vi "Create Live Random Data.vi"(0 "Input AnchorArray":refnum<class "Anchor.lvclass">[](array[class]), 7 "Tag.lvclass":refnum<class "Tag.lvclass">, 11 "Input":T3) -> (4 "PositionOut":T1, 8 "Output AnchorArray":refnum<class "Anchor.lvclass">[](array[class]), 15 "Output Tag":refnum<class "Tag.lvclass">)   [LabVIEW 2014]
doc: "This VI create random generated data based on its previous input, an array of Anchor objects and a single Tag object which we want its position estimated. The VI returns the Tag id, estimated position, and the altered array of Anchor objects. DistanceLimit control manages the limit on measured distances. If the measured distance >= DistanceLimit the distance is set to an invalid number so it will not be taken into account for position estimation. This control serves to simulate real world scenario where a signal can be lost\nafter a certain amount of meters."
uses:
  Tag.lvclass
  Anchor/Anchor.lvclass
panel:
  in  "DistanceLimit":dbl=90.0
  out "Tag out":refnum<class "Tag.lvclass">
  out "error out 2":errorcluster
  in  "error in (no error) 2":errorcluster
  out "error out":errorcluster
  in  "error in (no error)":errorcluster
  out "AnchorIDDistanceCluster":T2
  out "NumberOfAnchors":i32
  out "AnchorClusterArray":T4(array[cluster])
  out "TagY":dbl
  out "TagX":dbl
  out "TagID":dbl
  out "x rand":dbl
  out "y rand":dbl
  out "Start y":dbl=30.0
  out "Start x":dbl=61.0
  # "Use dynamic anchor array for multiple anchors.\nStandard is 3 anchors."
  # "Result of Create Random XY VI\nCompare with output for analysis"
  # "[tagID, x, y, anchorID, distances]"
  # "tagID, X, Y, [anchorID, distance]"
  # "Tag which has updated XY values"
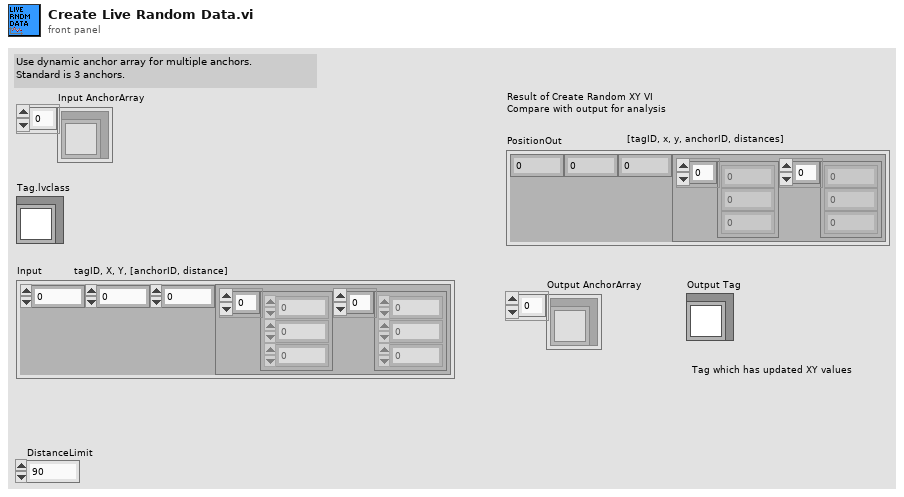
[diagram p1: front panel]
types:
  T1 = cluster{"tagID":dbl, "X":dbl, "Y":dbl, "anchorIDDistanceCluster":cluster{"anchorIDArray":dbl[], "anchorDistanceArray":dbl[]}}
  T2 = cluster{"AnchorIDArrayConstant":dbl[], "AnchorDistanceConstant":dbl[]}
  T3 = cluster{"Tag":dbl, "X":dbl, "Y":dbl, "AnchorIDDistanceCluster":cluster{"AnchorIDArray":dbl[], "AnchorDistancesArray":dbl[]}}
  T4 = cluster{"AnchorID":dbl, "AnchorX":dbl, "AnchorY":dbl}[]
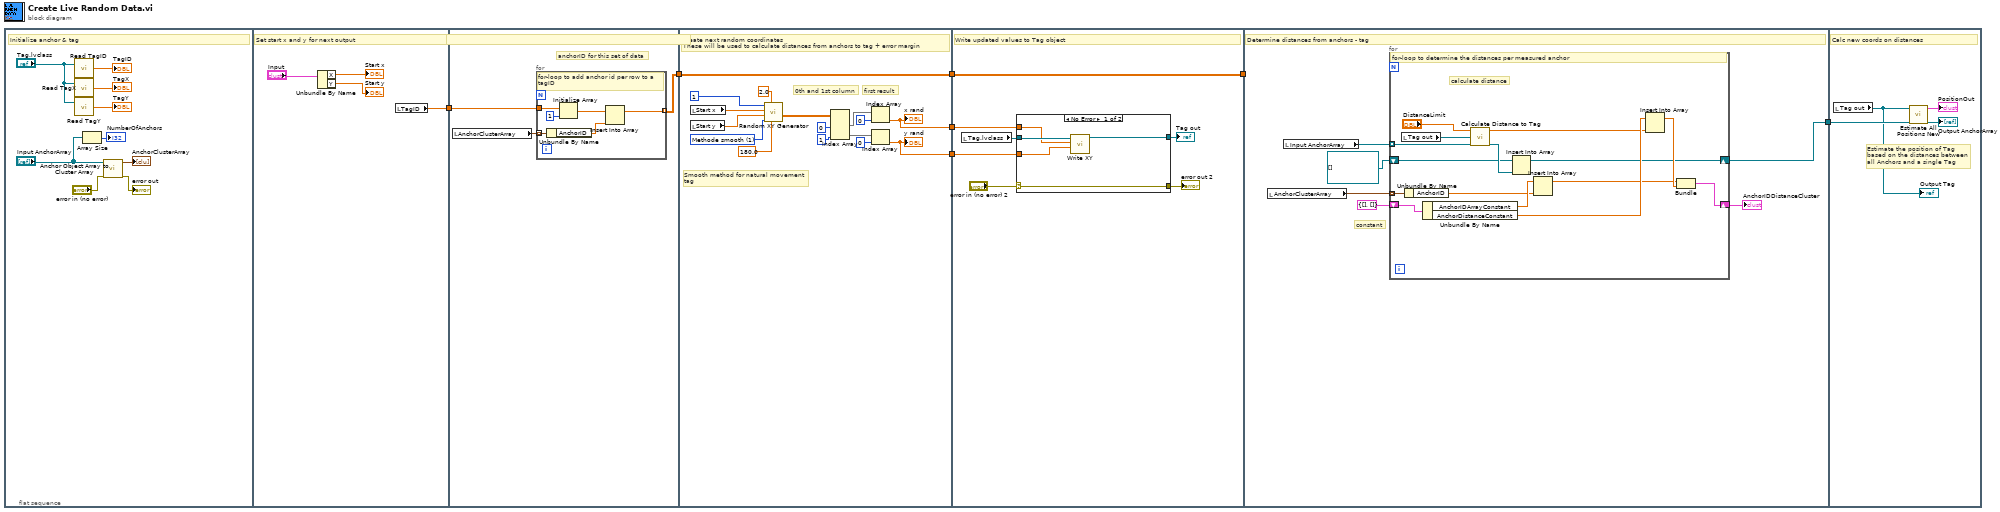
[diagram p0: block diagram]
diagram:
  n1 = flat-sequence {
    tunnel: [w20] -> w6
    tunnel: [w21] -> w7
    tunnel: w6 -> [w23]
    tunnel: [w45] -> w4
    tunnel: w7 -> [w45]
    tunnel: [w31] -> w2
    tunnel: [w30] -> w1
    tunnel: w4 -> [w52]
    tunnel: [w52] -> w3
    tunnel: w2 -> [w50]
    tunnel: w1 -> [w49]
    tunnel: w3 -> [_]
    tunnel: [w60] -> w5
    tunnel: w5 -> [w84]
    frame #0 {
      # "Initialize anchor & tag"
      n2 = call-dynamic "Read TagID.vi"("Tag in"="Tag.lvclass") -> ("TagID"=→"TagID":dbl)  [unwired: 1 in, 2 out]
      n3 = call-dynamic "Read TagX.vi"("Tag in"="Tag.lvclass") -> ("TagX"=→"TagX":dbl)  [unwired: 1 in, 2 out]
      n4 = call-dynamic "Read TagY.vi"("Tag in"="Tag.lvclass") -> ("TagY"=→"TagY":dbl)  [unwired: 1 in, 2 out]
      n5 = Array Size(array="Input AnchorArray") -> (size(s)=→"NumberOfAnchors":i32)
      n6 = call "Anchor Object Array to Cluster Array.vi"("error in (no error)"="error in (no error)", "AnchorArray In"="Input AnchorArray") -> ("error out"=→"error out":errorcluster, "AnchorArray Out"=→"AnchorClusterArray":T4)  [unwired: 8 in]
    }
    frame #1 {
      # "Set start x and y for next output"
      n7 = Unbundle By Name("Input") -> ("X"=→"Start x":dbl, "Y"=→"Start y":dbl)
      n8 = local read "TagID"() -> (w20:dbl)
    }
    frame #2 {
      # "anchorID for this set of data"
      # "Create anchor IDs"
      n9 = local read "AnchorClusterArray"() -> (w22:T4)
      n10 = for {
        tunnel: w23 -> [w28]
        tunnel: w22 -> [w29] mode=indexing
        tunnel: [w24] -> w21 mode=indexing
        # "for-loop to add anchor id per row to a tagID"
        n11 = Unbundle By Name(w29) -> ("AnchorID"=w25:dbl)
        n12 = Initialize Array ("Initialize Tag ID Row Array")(w28, 1 ("dimension size")) -> (w26:dbl[])
        n13 = Insert Into Array(array=w26, new element=w25) -> (w24:dbl[])  [unwired: 1 in]
      }
    }
    frame #3 {
      w44 = u16 1 items=["Methode Random", "Methode smooth"] ("Random Methode")
      # "first result"
      # "0th and 1st column"
      # "Smooth method for natural movement\ntag"
      # "Create next random coordinates\nThese will be used to calculate distances from anchors to tag + error margin"
      n14 = local read "Start x"() -> (w42:dbl)
      n15 = local read "Start y"() -> (w43:dbl)
      n16 = call "Random XY Generator.vi"("MaxHeading"=180.0 ("Max h variatie"), "MaxVelocity"=2.0 ("Max V variatie"), "Random Methode"=w44, "Y start"=w43, "X start"=w42, "number of rounds"=1) -> ("Array"=w38:dbl[][])  [unwired: 3 out]
      n17 = Index Array(array=w38, index (col) #1=0 ("disabled index (col)"), index (col) #2=1 ("index (col)")) -> (element #1=w35:dbl[], element #2=w34:dbl[])  [unwired: 2 in]
      n18 = Index Array(array=w35, index=0) -> (element=w31:dbl)
      "x rand" <- w31
      n19 = Index Array(array=w34, index=0) -> (element=w30:dbl)
      "y rand" <- w30
    }
    frame #4 {
      # "Write updated values to Tag object"
      n20 = local read "Tag.lvclass"() -> (w51:refnum<class "Tag.lvclass">)
      n21 = case shown="No Error" "error in (no error) 2" {
        selector: "error in (no error) 2" -> [w57 w59]
        tunnel: w51 -> [w56 w58]
        tunnel: w50 -> [w55 _]
        tunnel: w49 -> [w54 _]
        tunnel: [w57 w59] -> w47
        tunnel: [w53 w58] -> w46
        frame No Error {
          n22 = call "Write XY.vi"("TagY"=w54, "TagX"=w55, "Tag.lvclass"=w56) -> ("Tag Out"=w53:refnum<class "Tag.lvclass">)  [unwired: 7 in, 1 out]
        }
        frame Error {
        }
      }
      "error out 2" <- w47
      "Tag out" <- w46
    }
    frame #5 {
      # "constant"
      # "Determine distances from anchors - tag"
      n23 = local read "AnchorClusterArray"() -> (w65:T4)
      n24 = local read "Input AnchorArray"() -> (w62:refnum<class "Anchor.lvclass">[])
      n25 = for {
        tunnel: w65 -> [w80] mode=indexing
        shift-right: [w73] -> w63
        shift-left: T2 {"AnchorIDArrayConstant"=[], "AnchorDistanceConstant"=[]} ("AnchorIDDistanceClusterConstant") -> [w79]
        tunnel: w62 -> [w72] mode=indexing
        shift-right: [w69] -> w60
        shift-left: refnum<class "Anchor.lvclass">[] [] -> [w70]
        # "calculate distance"
        # "for-loop to determine the distances per measured anchor"
        n26 = local read "Tag out"() -> (w67:refnum<class "Tag.lvclass">)
        n27 = Unbundle By Name(w80) -> ("AnchorID"=w77:dbl)
        n28 = Unbundle By Name(w79) -> ("AnchorIDArrayConstant"=w78:dbl[], "AnchorDistanceConstant"=w76:dbl[])
        n29 = call "Calculate Distance to Tag.vi"("Anchor.lvclass In"=w72, "Tag.lvclass"=w67, "DistanceLimit"="DistanceLimit") -> ("Anchor out"=w71:refnum<class "Anchor.lvclass">, "Distance"=w68:dbl)  [unwired: 7 in]
        n30 = Insert Into Array(array=w70, new element=w71) -> (w69:refnum<class "Anchor.lvclass">[])  [unwired: 1 in]
        n31 = Insert Into Array(array=w78, new element=w77) -> (w74:dbl[])  [unwired: 1 in]
        n32 = Insert Into Array(array=w76, new element=w68) -> (w75:dbl[])  [unwired: 1 in]
        n33 = Bundle("AnchorIDArrayConstant"=w74, "AnchorDistanceConstant"=w75) -> (w73:T2)  [unwired: 1 in]
      }
      "AnchorIDDistanceCluster" <- w63
    }
    frame #6 {
      # "Estimate the position of Tag \nbased on the distances between\nall Anchors and a single Tag"
      # "Calc new coords on distances"
      n34 = local read "Tag out"() -> (w81:refnum<class "Tag.lvclass">)
      "Output Tag" <- w81
      n35 = call "Estimate All Positions New.vi"("Input AnchorArray"=w84, "Tag.lvclass"=w81) -> ("Output AnchorArray"=→"Output AnchorArray":refnum<class "Anchor.lvclass">[], "PositionCluster [tagID, x, y, anchorID, distances]"=→"PositionOut":T1)  [unwired: 8 in]
    }
  }
